vi "Execute (2D string).vi"(8 "error in (no error)":errorcluster, 10 "command":string, 11 "PQ Connection in":refnum<class "PQ Connection.lvclass">) -> (0 "error out":errorcluster, 1 "Strings":string[][](array[string]), 3 "PQ Connection out":refnum<class "PQ Connection.lvclass">)   [LabVIEW 2016, in "PQ Connection.lvclass"]
uses:
  PQ Connection.lvclass
  Result/PQ Result.lvclass
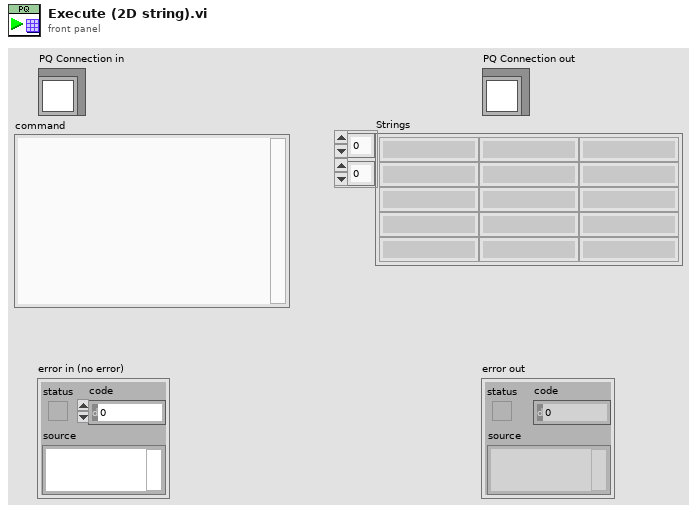
[diagram p1: front panel]
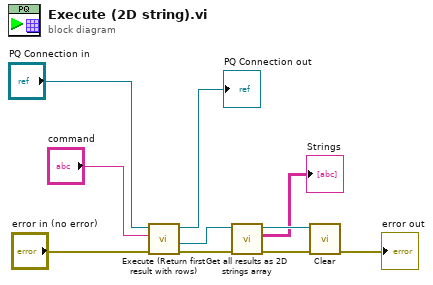
[diagram p0: block diagram]
diagram:
  n1 = call "Execute (Return first result with rows).vi"("error in (no error)"="error in (no error)", "SQL"="command", "PQ Connection in"="PQ Connection in") -> ("error out"=w4:errorcluster, "First Result with Rows returned"=w7:refnum<class "PQ Result.lvclass">, "PQ Connection out"=→"PQ Connection out":refnum<class "PQ Connection.lvclass">)  [unwired: 5 in, 1 out]
  n2 = call "Get all results as 2D strings array.vi"("error in (no error)"=w4, "PQ Result in"=w7) -> ("error out"=w5:errorcluster, "Strings"=→"Strings":string[][], "PQ Result out"=w6:refnum<class "PQ Result.lvclass">)  [unwired: 7 in]
  n3 = call "Clear.vi"("error in (no error)"=w5, "PQ Result  in"=w6) -> ("error out"=→"error out":errorcluster)  [unwired: 9 in]
